vi "Get Database Connection.vi"() -> (1 "Database  Connection String":string)   [LabVIEW 2018]
uses:
  <vilib>/Utility/config.llb/Read Key (String).vi
  <vilib>/Utility/config.llb/NI_LVConfig.lvlib
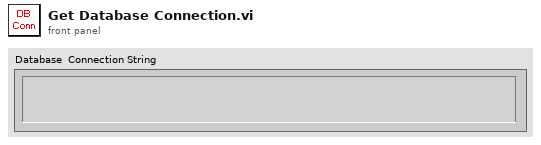
[diagram p1: front panel]
types:
  T1 = typedef "NI_LVConfig.lvlib/Config Data RefNum.ctl" = refnum<k1>
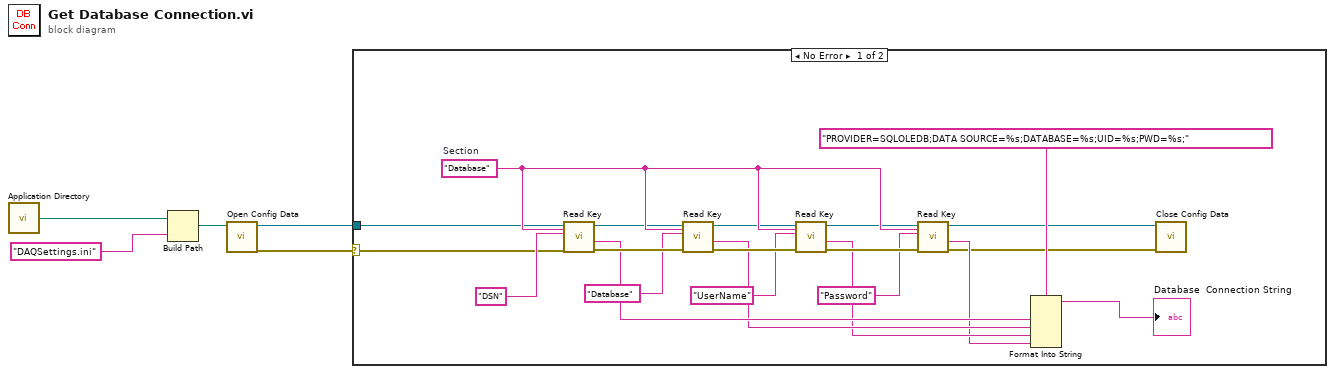
[diagram p0: block diagram]
diagram:
  n1 = call <vilib>:"Application Directory.vi"() -> ("Application Directory"=w5:path)
  n2 = Build Path(base path=w5, name or relative path="DAQSettings.ini") -> (appended path=w3:path)
  n3 = call <vilib>:"Open Config Data.vi"("configuration file path"=w3) -> ("error out"=w1:errorcluster, "refnum"=w2:T1)  [unwired: 8 in, 1 out]
  n4 = case shown="No Error" w1 {
    selector: w1 -> [w7 _]
    tunnel: w2 -> [w8 _]
    frame No Error {
      w26 = "Database"  # Section
      n5 = call-poly <vilib>:"Read Key.vi"("section"=w26, "error in (no error)"=w7, "key"="DSN", "refnum"=w8) -> ("error out"=w17:errorcluster, "value"=w14:string, "refnum out"=w18:T1)  [unwired: 4 in, 1 out]
      n6 = call-poly <vilib>:"Read Key.vi"("section"=w26, "error in (no error)"=w17, "key"="Database", "refnum"=w18) -> ("error out"=w23:errorcluster, "value"=w13:string, "refnum out"=w22:T1)  [unwired: 4 in, 1 out]
      n7 = call-poly <vilib>:"Read Key.vi"("section"=w26, "error in (no error)"=w23, "key"="UserName", "refnum"=w22) -> ("error out"=w25:errorcluster, "value"=w12:string, "refnum out"=w24:T1)  [unwired: 4 in, 1 out]
      n8 = call-poly <vilib>:"Read Key.vi"("section"=w26, "error in (no error)"=w25, "key"="Password", "refnum"=w24) -> ("error out"=w9:errorcluster, "value"=w11:string, "refnum out"=w10:T1)  [unwired: 4 in, 1 out]
      n9 = Format Into String(format string="PROVIDER=SQLOLEDB;DATA SOURCE=%s;DATABASE=%s;UID=%s;PWD=%s;", w14, w13, w12, w11) -> (resulting string=→"Database  Connection String":string)  [unwired: 2 in, 1 out]
      n10 = call <vilib>:"Close Config Data.vi"("error in (no error)"=w9, "refnum"=w10) -> ()  [unwired: 8 in, 2 out]
    }
    frame Error {
    }
  }
